vi "Example 5 - SubVIs.vi"   [LabVIEW 2015]
uses:
  library/Scripting.lvlib
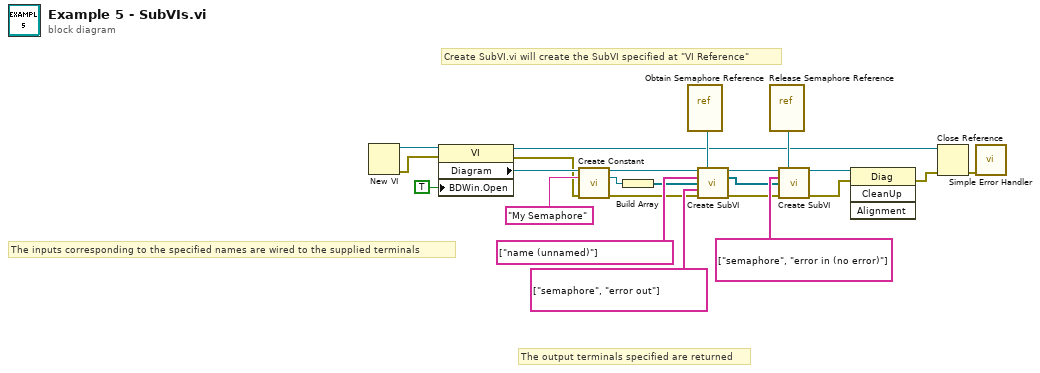
[diagram p0: block diagram]
diagram:
  # "The output terminals specified are returned"
  # "The inputs corresponding to the specified names are wired to the supplied terminals"
  # "Create SubVI.vi will create the SubVI specified at \"VI Reference\""
  n1 = New VI() -> (0:w19:errorcluster, 3:w20:refnum<vi>)  [unwired: 7 in]
  n2 = property class="VI"(reference=w20, error in=w19, "BDWin.Open"=TRUE ("Block Diagram Window:Open")) -> (reference out=w1:refnum<vi>, error out=w16:errorcluster, "Diagram"=w17:refnum<vi>)
  n3 = call "Create Constant.vi"("Diagram in"=w17, "Type"="My Semaphore", "error in (no error)"=w16) -> ("Diagram out"=w14:refnum<vi>, "Terminal"=w11:refnum<vi>, "error out"=w9:errorcluster)  [unwired: 10 in]
  n4 = Build Array(w11) -> (w10:refnum<vi>[])
  n5 = vi-ref <vilib>:"Obtain Semaphore Reference.vi"() -> (w15:refnum<vi>)
  n6 = call "Create SubVI.vi"("Diagram in"=w14, "VI Reference"=w15, "Input Names"=string[] ["name (unnamed)"], "Inputs"=w10, "Output Names"=string[] ["semaphore", "error out"] ("Input Names"), "error in (no error)"=w9) -> ("Diagram out"=w7:refnum<vi>, "Outputs"=w5:refnum<vi>[], "error out"=w4:errorcluster)  [unwired: 7 in]
  n7 = vi-ref <vilib>:"Release Semaphore Reference.vi"() -> (w8:refnum<vi>)
  n8 = call "Create SubVI.vi"("Diagram in"=w7, "VI Reference"=w8, "Input Names"=string[] ["semaphore", "error in (no error)"], "Inputs"=w5, "error in (no error)"=w4) -> ("Diagram out"=w3:refnum<vi>, "error out"=w2:errorcluster)  [unwired: 8 in, 1 out]
  n9 = invoke class="Diag" method="CleanUp"(reference=w3, error in=w2) -> (error out=w22:errorcluster)  [unwired: 2 in, 3 out]
  n10 = Close Reference(reference=w1, error in (no error)=w22) -> (error out=w21:errorcluster)
  n11 = call <vilib>:"Simple Error Handler.vi"("error in (no error)"=w21) -> ()  [unwired: 4 in, 5 out]
